vi "ComponentSimulator.vi"(8 "error in":errorcluster) -> (0 "error out":errorcluster)   [LabVIEW 2018]
doc: "Simulate a software component that will use the Tcp Server."
uses:
  src/TcpServer/TcpServer.lvclass
  src/TcpServer/typedef/tcpPacketTypeDef.ctl
  src/TcpServer/typedef/eventTypeDef.ctl
  src/TcpServer/runServer.vi
panel:
  out "JSON Packet Received":string
  in  "Tab Control":T1(tab)
  out "confData":T2={"serverPort"=8888, "serverTimeout (ms)"=100, "serverBytesToRead"=32768} caption="Server Configurations"
  in  "fail":bool
  in  "success":bool
  in  "send_event":bool
  in  "evtName":string="move" caption="Event Name"
  in  "Event Details":string="\"InPosition\" : true\n\n\"Tolerance\" : 0.2"
  in  "stop_server":bool
  in  "Stop Simulator":bool caption="stop"
  # "Component Simulator"
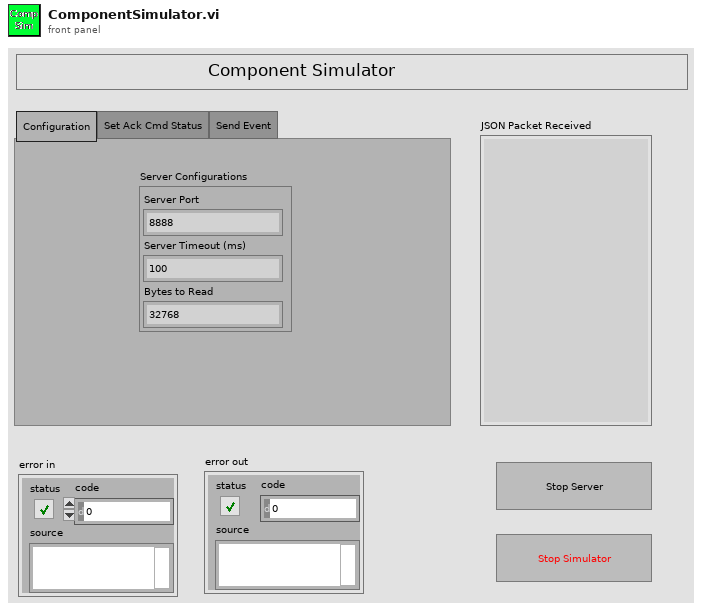
[diagram p1: front panel]
types:
  T1 = enum32{"Configuration", "Set Ack Cmd Status", "Send Event"}
  T2 = cluster{"serverPort":u16, "serverTimeout (ms)":i32, "serverBytesToRead":i32}
  T3 = typedef "TcpServer.lvclass/tcpPacketTypeDef.ctl" = cluster{"packet":string, "firstPacket":bool, "firstConnection":bool}
  T4 = typedef "TcpServer.lvclass/eventTypeDef.ctl" = cluster{"evtName":string, "evtDetails":string}
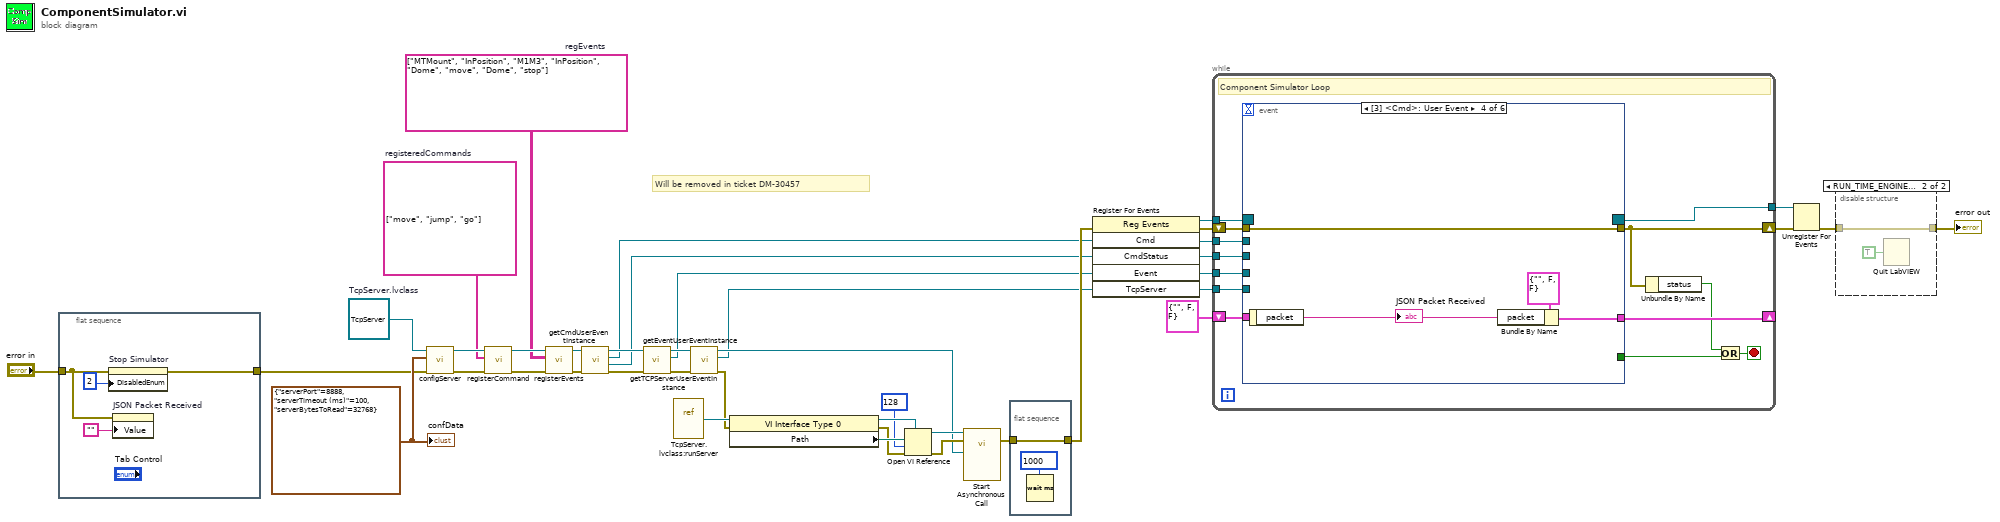
[diagram p0: block diagram]
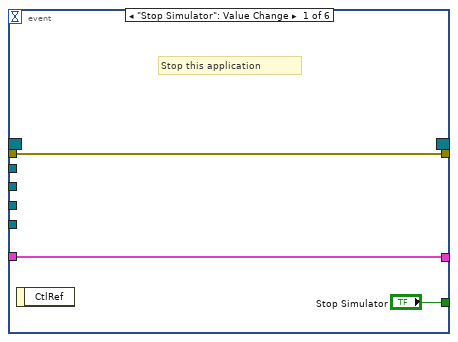
[diagram p3: hidden frame]
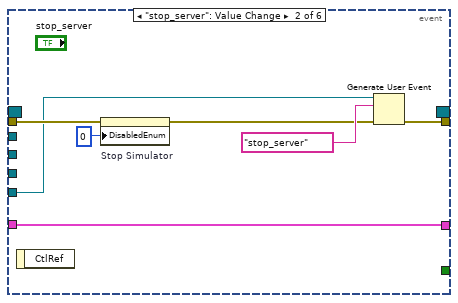
[diagram p4: hidden frame]
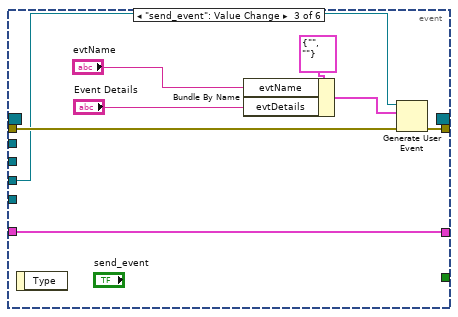
[diagram p5: hidden frame]
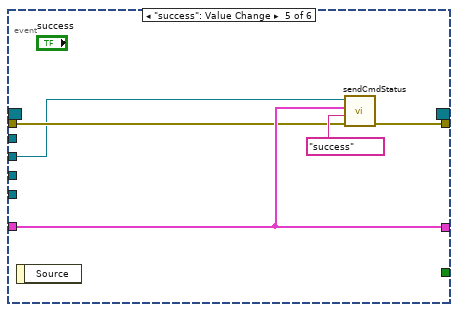
[diagram p6: hidden frame]
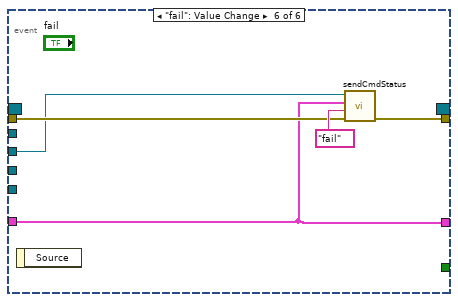
[diagram p7: hidden frame]
diagram:
  w1 = string[][] [["MTMount", "InPosition"], ["M1M3", "InPosition"], ["Dome", "move"], ["Dome", "stop"]]  # regEvents
  w31 = string[] ["move", "jump", "go"]  # registeredCommands
  w30 = T2 {"serverPort"=8888, "serverTimeout (ms)"=100, "serverBytesToRead"=32768} ("confData")
  w35 = refnum<class "TcpServer.lvclass"> refnum  # TcpServer.lvclass
  # "Will be removed in ticket DM-30457"
  n1 = flat-sequence {
    tunnel: "error in" -> [w40]
    tunnel: [w41] -> w5
    frame #0 {
      n2 = property on="Stop Simulator" class="Bool"(error in=w40, "DisabledEnum"=2) -> (error out=w41:errorcluster)  [unwired: 1 in, 1 out]
      n3 = property on="JSON Packet Received" class="Str"(error in=w40, "Value"="") -> ()  [unwired: 1 in, 2 out]
    }
  }
  n4 = call "configServer.vi"("error in (no error)"=w5, "confData"=w30, "tcpServer in"=w35) -> ("error out"=w34:errorcluster, "tcpServer out"=w32:refnum<class "TcpServer.lvclass">)  [unwired: 7 in]
  n5 = call "registerCommand.vi"("error in (no error)"=w34, "registeredCommands"=w31, "tcpServer in"=w32) -> ("error out"=w33:errorcluster, "tcpServer out"=w3:refnum<class "TcpServer.lvclass">)  [unwired: 7 in]
  n6 = call "registerEvents.vi"("error in (no error)"=w33, "registeredEvents"=w1, "tcpServer in"=w3) -> ("error out"=w4:errorcluster, "tcpServer out"=w2:refnum<class "TcpServer.lvclass">)  [unwired: 7 in]
  n7 = call "getCmdUserEventInstance.vi"("error in (no error)"=w4, "tcpServer in"=w2) -> ("error out"=w29:errorcluster, "CmdStatus"=w9:refnum<user-event>, "Cmd"=w10:refnum<user-event>, "tcpServer out"=w27:refnum<class "TcpServer.lvclass">)  [unwired: 6 in]
  n8 = call "getEventUserEventInstance.vi"("error in (no error)"=w29, "tcpServer in"=w27) -> ("error out"=w28:errorcluster, "Event"=w8:refnum<user-event>, "tcpServer out"=w26:refnum<class "TcpServer.lvclass">)  [unwired: 7 in]
  n9 = vi-ref "TcpServer.lvclass:runServer.vi"() -> (w25:refnum<vi>)
  n10 = call "getTCPServerUserEventInstance.vi"("error in (no error)"=w28, "tcpServer in"=w26) -> ("error out"=w18:errorcluster, "TcpServer"=w7:refnum<user-event>, "tcpServer out"=w17:refnum<class "TcpServer.lvclass">)  [unwired: 7 in]
  n11 = property class="VI Interface Type 0"(reference=w25, error in=w18) -> (reference out=w23:refnum<vi>, error out=w20:errorcluster, "Path"=w24:path)
  n12 = Open VI Reference(type specifier VI Refnum (for type only)=w23, vi path=w24, options=128, error in (no error)=w20) -> (vi reference=w21:refnum<vi>, error out=w19:errorcluster)  [unwired: 2 in]
  n13 = call-by-ref "Start Asynchronous Call"(reference=w21, error in=w19, "TcpServer in"=w17) -> (error out=w16:errorcluster)  [unwired: 9 in, 3 out]
  n14 = flat-sequence {
    tunnel: w16 -> [w43]
    tunnel: [w43] -> w15
    frame #0 {
      n15 = Wait (ms)(milliseconds to wait=u32 1000) -> ()  [unwired: 1 out]
    }
  }
  n16 = register-events(error in=w15, w10, w9, w8, w7) -> (reference out=w37:refnum<event-registration>, error out=w36:errorcluster)  [unwired: 1 in]
  n17 = while {
    tunnel: w37 -> [w56]
    shift-right: [w55] -> _
    shift-left: T3 {"packet"="", "firstPacket"=FALSE, "firstConnection"=FALSE} ("packetConnID") -> [w54]
    shift-right: [w51] -> w14
    shift-left: w36 -> [w57]
    tunnel: [w49] -> w12
    tunnel: w10 -> [w48]
    tunnel: w9 -> [w47]
    tunnel: w8 -> [w46]
    tunnel: w7 -> [w45]
    stop <- w53 stop-if-true
    # "Component Simulator Loop"
    n18 = event shown="[3] <Cmd>: User Event" {
      selector: w56 -> [_ _ _ _ _ _]
      dyn-events: [_ _ _ _ _ _] -> w49
      timeout: _ -> [_ _ _ _ _ _]
      tunnel: ["Stop Simulator" _ _ _ _ _] -> w52
      tunnel: [w59 w65 w75 w79 w83 w88] -> w51
      tunnel: w57 -> [w59 w63 w74 w79 w81 w87]
      tunnel: [w58 w64 w72 w76 w82 w86] -> w55
      tunnel: w54 -> [w58 w64 w72 _ w82 w86]
      tunnel: w48 -> [_ _ _ _ _ _]
      tunnel: w47 -> [_ _ _ _ w80 w85]
      tunnel: w46 -> [_ _ w69 _ _ _]
      tunnel: w45 -> [_ w61 _ _ _ _]
      event "Stop Simulator": Value Change {
        # "Stop this application"
        n19 = event-data() -> ()  [unwired: 1 in, 1 out]
      }
      event "stop_server": Value Change {
        n20 = event-data() -> ()  [unwired: 1 in, 1 out]
        n21 = property on="Stop Simulator" class="Bool"(error in=w63, "DisabledEnum"=0) -> (error out=w62:errorcluster)  [unwired: 1 in, 1 out]
        n22 = Generate User Event(user event=w61, event data cluster="stop_server" ("event data"), error in=w62) -> (error out=w65:errorcluster)  [unwired: 1 in, 1 out]
      }
      event "send_event": Value Change {
        n23 = event-data() -> ()  [unwired: 1 in, 1 out]
        n24 = Bundle By Name(cluster=T4 {"evtName"="", "evtDetails"=""} ("eventConnID"), "evtName"="evtName", "evtDetails"="Event Details") -> (w70:T4)
        n25 = Generate User Event(user event=w69, event data cluster=w70, error in=w74) -> (error out=w75:errorcluster)  [unwired: 1 in, 1 out]
      }
      event User Event {
        n26 = event-data() -> ("packet"=w77:string)  [unwired: 1 in]
        "JSON Packet Received" <- w77
        n27 = Bundle By Name(cluster=T3 {"packet"="", "firstPacket"=FALSE, "firstConnection"=FALSE} ("packetConnID"), "packet"=w77) -> (w76:T3)
      }
      event "success": Value Change {
        n28 = event-data() -> ()  [unwired: 1 in, 1 out]
        n29 = call "sendCmdStatus.vi"("error in (no error)"=w81, "cmdStatus"="success", "packetConnID"=w82, "user event"=w80) -> ("error out"=w83:errorcluster)  [unwired: 7 in]
      }
      event "fail": Value Change {
        n30 = event-data() -> ()  [unwired: 1 in, 1 out]
        n31 = call "sendCmdStatus.vi"("error in (no error)"=w87, "cmdStatus"="fail", "packetConnID"=w86, "user event"=w85) -> ("error out"=w88:errorcluster)  [unwired: 7 in]
      }
    }
    n32 = Unbundle By Name(w51) -> ("status"=w50:bool)
    n33 = Or(x=w50, y=w52) -> (x .or. y?=w53:bool)
  }
  n34 = Unregister For Events(event registration refnum=w12, error in=w14) -> (error out=w13:errorcluster)
  n35 = disable-structure shown="RUN_TIME_ENGINE==True" {
    disable-tunnel: w13 -> [w90 w91]
    disable-tunnel: [w90 w91] -> w38
    frame condition #0 (active) {
    }
    frame condition #1 {
      n36 = Quit LabVIEW(quit? (T)=TRUE) -> ()
    }
  }
  "error out" <- w38
  "confData" <- w30
